vi "Logged_Data_Global.vi"(2 "Data In":dbl[][](array[numeric]) format="%.2f", 3 "Set Global":bool) -> (0 "Data Out":dbl[][](array[numeric]) format="%.2f", 1 "Valid?":bool)   [LabVIEW 2010]
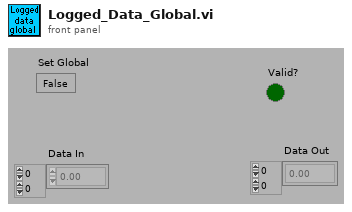
[diagram p1: front panel]
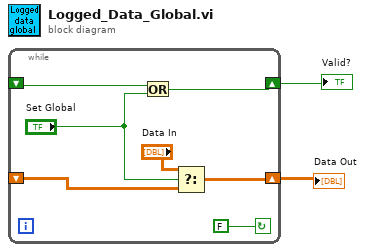
[diagram p0: block diagram]
diagram:
  n1 = while {
    shift-left: _ -> [w4]
    shift-right: [w5] -> w1
    shift-left: _ -> [w9]
    shift-right: [w8] -> w2
    stop <- FALSE continue-if-true
    n2 = Or(x=w9, y="Set Global") -> (x .or. y?=w8:bool)
    n3 = Select(t="Data In", s="Set Global", f=w4) -> (s? t:f=w5:dbl[][])
  }
  "Data Out" <- w1
  "Valid?" <- w2
